vi "Channels Write.vi"(4 "error in (no error)":errorcluster, 5 "Value":string[](array[string]), 6 "Container State":T2, 7 "Display State In":T1 {"Time_data" format="%<%.3X>T"}) -> (0 "error out":errorcluster, 3 "Display State Out":T1 {"Time_data" format="%<%.3X>T"})   [LabVIEW 2019, in "2D Buffer Display.xctl"]
uses:
  2D Buffer Display.xctl
  <vilib>/_xctls/Container State.ctl
  Graph_State.ctl
  <vilib>/_xctls/XControlSupport.lvlib
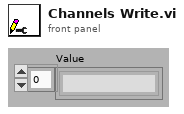
[diagram p1: front panel]
types:
  T1 = typedef "2D Buffer Display.xctl/Graph_State.ctl" = cluster{"History":u16, "Time_data":timestamp[], "Data_Out":sgl[][][], "Channels":bool[], "Variable":bool[], "Variable Tags":string[], "Channel Tags":string[], "Plot Details":cluster{"Name":string, "Line Width":u8, "Line Style":u8, "Color":u32}[], "Y-Axis Labels":string[], "Avg Data":cluster{"mean":dbl, "standard deviation":dbl}[][]}
  T2 = typedef "XControlSupport.lvlib/Container State.ctl" = cluster{"Indicator?":bool, "Run Mode?":bool, " Refnum":refnum<vi>}
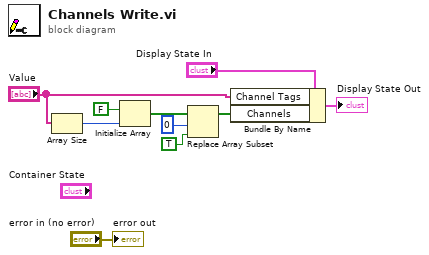
[diagram p0: block diagram]
diagram:
  n1 = Array Size(array="Value") -> (size(s)=w6:i32)
  n2 = Initialize Array(FALSE, w6) -> (w4:bool[])
  n3 = Replace Array Subset(array=w4, new element=TRUE, index=0) -> (w1:bool[])
  n4 = Bundle By Name(cluster="Display State In", "Channel Tags"="Value", "Channels"=w1) -> (→"Display State Out":T1)
  "error out" <- "error in (no error)"
